vi "HardwareOutput.vi"(8 "error in":errorcluster, 9 "Update Outputs":bool, 10 "Motor Control Cluster":T1, 11 "DAQREFs in":T3) -> (0 "error out":errorcluster, 3 "DAQREFs out":T3)   [LabVIEW 2021]
uses:
  controls/DAQ Refnums.ctl
  TypeDef/MotorControlCluster.ctl
  controls/Status Lights.ctl
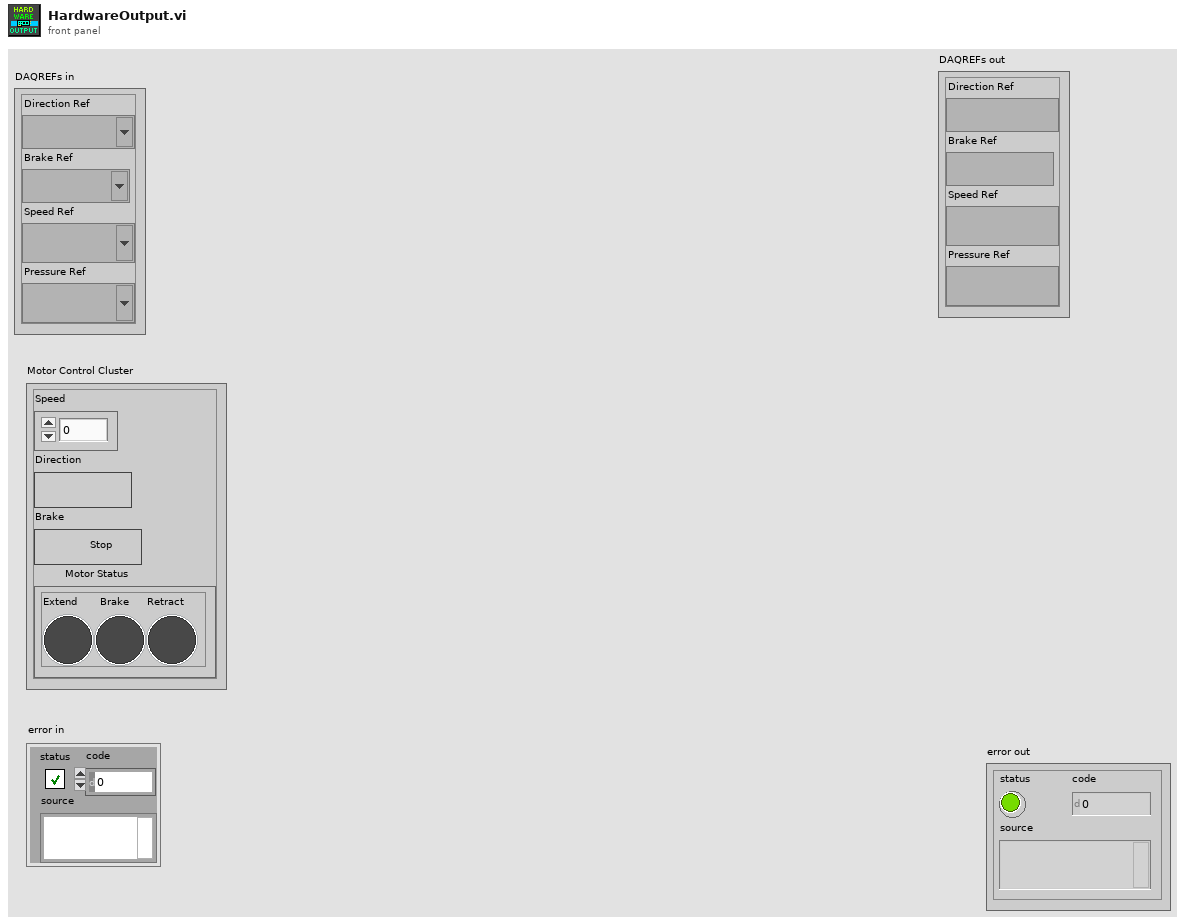
[diagram p1: front panel]
types:
  T1 = typedef "MotorControlCluster.ctl" = cluster{"Speed":dbl, "Direction":bool, "Brake":bool, "Motor Status":T2}
  T2 = typedef "Status Lights.ctl" = cluster{"Extend":bool, "Brake":bool, "Retract":bool}
  T3 = typedef "DAQ Refnums.ctl" = cluster{"Direction Ref":refnum<k21>, "Brake Ref":refnum<k21>, "Speed Ref":refnum<k21>, "Pressure Ref":refnum<k21>}
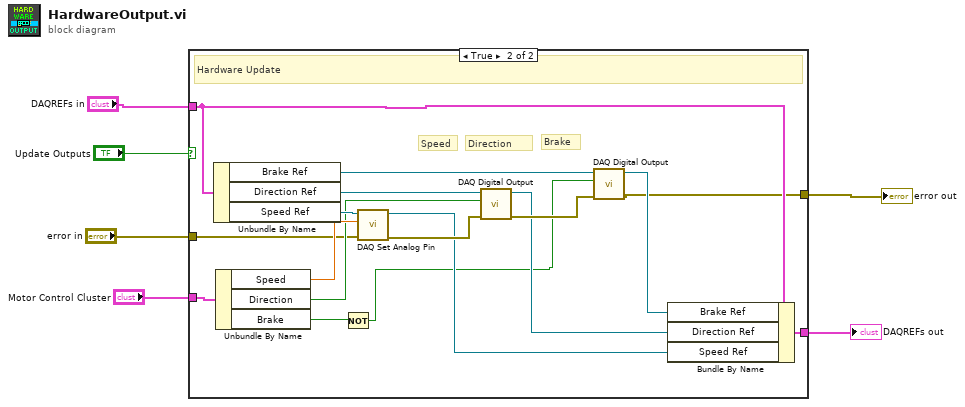
[diagram p0: block diagram]
diagram:
  n1 = case shown="True" "Update Outputs" {
    tunnel: "DAQREFs in" -> [w7 w22]
    tunnel: [w7 w23] -> w6
    tunnel: "Motor Control Cluster" -> [_ w15]
    tunnel: [w8 w12] -> w2
    tunnel: "error in" -> [w8 w11]
    frame False {
      # "No Hardware Update"
    }
    frame True {
      # "Brake"
      # "Direction"
      # "Speed"
      # "Hardware Update"
      n2 = Unbundle By Name(w22) -> ("Brake Ref"=w19:refnum<k21>, "Direction Ref"=w20:refnum<k21>, "Speed Ref"=w21:refnum<k21>)
      n3 = Unbundle By Name(w15) -> ("Speed"=w14:dbl, "Direction"=w13:bool, "Brake"=w10:bool)
      n4 = Not(x=w10) -> (.not. x?=w9:bool)
      n5 = call "DAQ Set Analog Pin.vi"("error in"=w11, "Voltage"=w14, "task/channels in"=w21) -> ("error out"=w25:errorcluster, "task out"=w18:refnum<k21>)  [unwired: 6 in, 1 out]
      n6 = call "DAQ Digital Output.vi"("error in"=w25, "data"=w13, "task/channels in"=w20) -> ("error out"=w24:errorcluster, "task out"=w17:refnum<k21>)  [unwired: 6 in, 1 out]
      n7 = call "DAQ Digital Output.vi"("error in"=w24, "data"=w9, "task/channels in"=w19) -> ("error out"=w12:errorcluster, "task out"=w16:refnum<k21>)  [unwired: 6 in, 1 out]
      n8 = Bundle By Name(cluster=w22, "Brake Ref"=w16, "Direction Ref"=w17, "Speed Ref"=w18) -> (w23:T3)
    }
  }
  "DAQREFs out" <- w6
  "error out" <- w2
